vi "GetAdapters.vi"(8 "error in":errorcluster) -> (0 "error out":errorcluster, 3 "AdaptersOut":T1[](array[typedef]))   [LabVIEW 2011, in "Konvolucio MCAN120803.lvlib"]
doc: "Specifies the list of adapters connected to a Host."
uses:
  <instrlib>/Konvolucio MCAN120803/Konvolucio MCAN120803.lvlib
  <instrlib>/Konvolucio MCAN120803/Types/AdapterItemType.ctl
  C:/Program Files/National Instruments/LabVIEW 2011/instr.lib/Konvolucio MCAN120803/Private/Konvolucio.MCAN120803.API.dll
  Private/Konvolucio.MCAN120803.API.dll
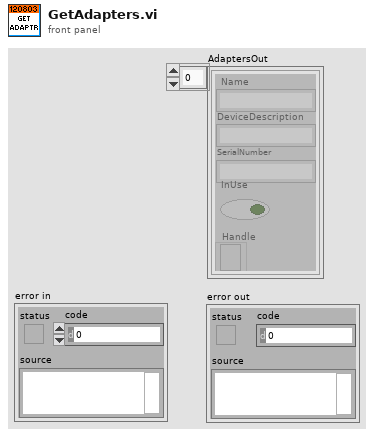
[diagram p1: front panel]
types:
  T1 = typedef "Konvolucio MCAN120803.lvlib/AdapterItemType.ctl" = cluster{"Name":string, "DeviceDescription":string, "SerialNumber":string, "InUse":bool, "Handle":refnum<k24>}
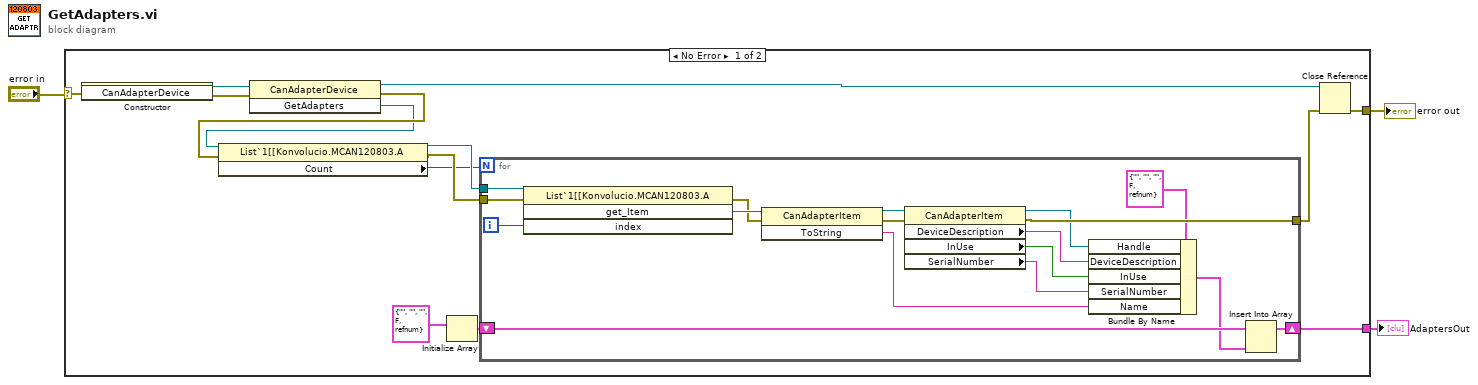
[diagram p0: block diagram]
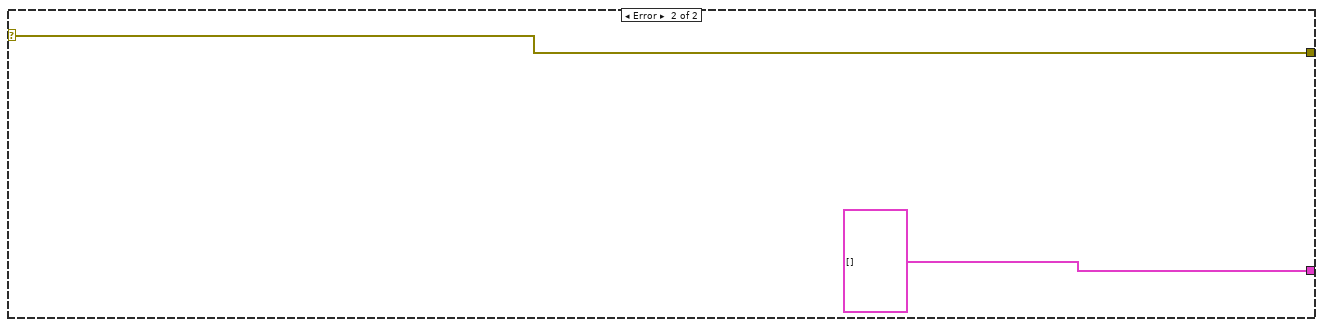
[diagram p2: hidden frame]
diagram:
  n1 = case shown="No Error" "error in" {
    selector: "error in" -> [w13 w35]
    tunnel: [w15 T1[] []] -> w3
    tunnel: [w14 w35] -> w2
    frame No Error {
      n2 = constructor class="CanAdapterDevice" ("MCanAdapter")(error in=w13) -> (reference out=w10:refnum<k24>, error out=w9:errorcluster)  [unwired: 2 in, 1 out]
      n3 = invoke class="CanAdapterDevice" method="GetAdapters"(reference=w10, error in=w9) -> (reference out=w11:refnum<k24>, error out=w8:errorcluster, "GetAdapters"=w4:refnum<k24>)  [unwired: 1 in]
      n4 = property class="List`1[[Konvolucio.MCAN120803.A"(reference=w4, error in=w8) -> (reference out=w7:refnum<k24>, error out=w6:errorcluster, "Count"=w5:i32)
      n5 = Initialize Array(T1 {"Name"="", "DeviceDescription"="", "SerialNumber"="", "InUse"=FALSE, "Handle"=refnum}) -> (w16:T1[])  [unwired: 1 in]
      n6 = for {
        N: w5 -> [_]
        tunnel: w6 -> [w31]
        shift-right: [w33] -> w15
        shift-left: w16 -> [w34]
        tunnel: w7 -> [w30]
        tunnel: [w20] -> w12
        i -> [w29]
        n7 = invoke class="List`1[[Konvolucio.MCAN120803.A" method="get_Item"(reference=w30, error in=w31, "index"=w29) -> (error out=w27:errorcluster, "get_Item"=w28:refnum<k24>)  [unwired: 1 in, 2 out]
        n8 = invoke class="CanAdapterItem" method="ToString"(reference=w28, error in=w27) -> (reference out=w25:refnum<k24>, error out=w24:errorcluster, "ToString"=w26:string)  [unwired: 1 in]
        n9 = property class="CanAdapterItem"(reference=w25, error in=w24) -> (reference out=w18:refnum<k24>, error out=w20:errorcluster, "DeviceDescription"=w21:string, "InUse"=w22:bool, "SerialNumber"=w23:string)
        n10 = Bundle By Name(cluster=T1 {"Name"="", "DeviceDescription"="", "SerialNumber"="", "InUse"=FALSE, "Handle"=refnum} ("AdapterItemType"), "Handle"=w18, "DeviceDescription"=w21, "InUse"=w22, "SerialNumber"=w23, "Name"=w26) -> (w32:T1)
        n11 = Insert Into Array(array=w34, new element=w32) -> (w33:T1[])  [unwired: 1 in]
      }
      n12 = Close Reference(reference=w11, error in (no error)=w12) -> (error out=w14:errorcluster)
    }
    frame Error {
    }
  }
  "AdaptersOut" <- w3
  "error out" <- w2
